vi "FloaterThreshAverage.vi"() -> ()   [LabVIEW 2022 SP3]
uses:
  <vilib>/Utility/file.llb/Read Delimited Spreadsheet (string).vi
panel:
  out "Array":string[][](array[string])
  in  "new path in":path=path "E:/Vitreous/CUMC/Single Element/SingleFloatersCompiled/AA_ThreshMaskResults.txt"
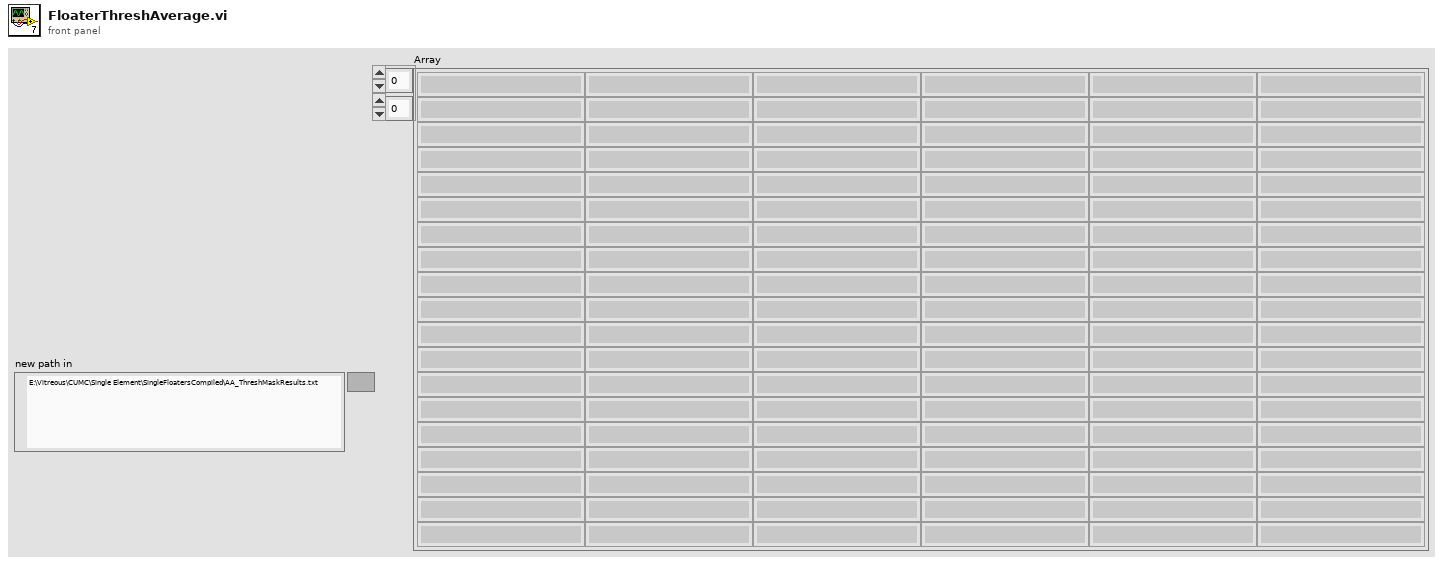
[diagram p1: front panel]
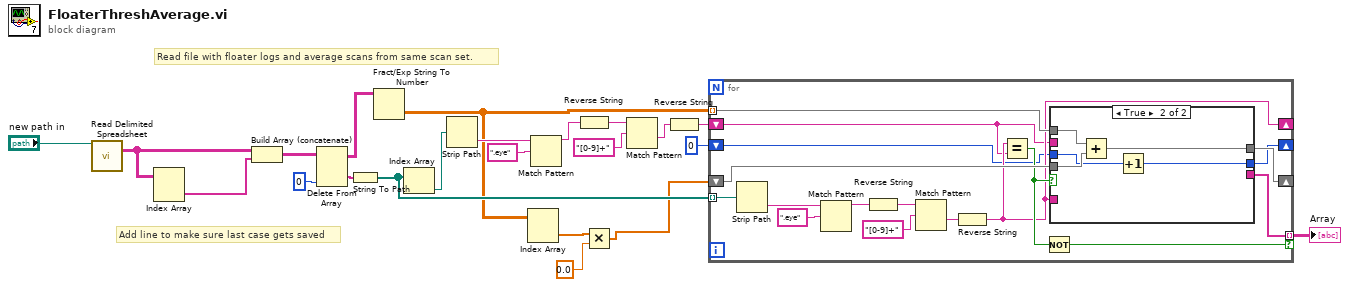
[diagram p0: block diagram]
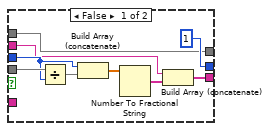
[diagram p2: hidden frame]
diagram:
  # "Read file with floater logs and average scans from same scan set."
  # "Add line to make sure last case gets saved"
  n1 = call-poly <vilib>:"Read Delimited Spreadsheet.vi"("file path (dialog if empty)"="new path in") -> ("all rows"=w2:string[][])  [unwired: 9 in, 5 out]
  n2 = Index Array(array=w2) -> (element=w1:string[])  [unwired: 2 in]
  n3 = Build Array (concatenate)(w2, w1) -> (w7:string[][])
  n4 = Delete From Array(array=w7, index (col)=0 ("index (row)")) -> (deleted portion=w8:string[], array with subset deleted=w20:string[][])  [unwired: 2 in]
  n5 = String To Path(string=w8) -> (path=w12:path[])
  n6 = Fract/Exp String To Number(string=w20) -> (number=w6:dbl[][])  [unwired: 3 in, 1 out]
  n7 = Index Array(array=w12) -> (element=w11:path)  [unwired: 1 in]
  n8 = Strip Path(path=w11) -> (name=w10:string)  [unwired: 1 out]
  n9 = Index Array(array=w6) -> (element=w5:dbl[])  [unwired: 2 in]
  n10 = Match Pattern(string=w10, regular expression=".eye") -> (before substring=w16:string)  [unwired: 1 in, 3 out]
  n11 = Reverse String(1:w16) -> (0:w15:string)
  n12 = Multiply(x=w5, y=0.0) -> (x*y=w4:dbl[])
  n13 = Match Pattern(string=w15, regular expression="[0-9]+") -> (after substring=w13:string)  [unwired: 1 in, 3 out]
  n14 = Reverse String(1:w13) -> (0:w9:string)
  n15 = for {
    tunnel: w12 -> [w39] mode=indexing
    shift-right: [w25] -> _
    shift-left: w9 -> [w23]
    tunnel: w6 -> [w32] mode=indexing
    shift-right: [w31] -> _
    shift-left: w4 -> [w30]
    shift-right: [w29] -> _
    shift-left: i16 0 -> [w24]
    tunnel: [w26] -> w18 mode=indexing if=w27
    n16 = Strip Path(path=w39) -> (name=w37:string)  [unwired: 1 out]
    n17 = Match Pattern(string=w37, regular expression=".eye") -> (before substring=w36:string)  [unwired: 1 in, 3 out]
    n18 = Reverse String(1:w36) -> (0:w35:string)
    n19 = Match Pattern(string=w35, regular expression="[0-9]+") -> (after substring=w33:string)  [unwired: 1 in, 3 out]
    n20 = Reverse String(1:w33) -> (0:w25:string)
    n21 = Equal?(x=w25, y=w23) -> (x = y?=w28:bool)
    n22 = Not(x=w28) -> (.not. x?=w27:bool)
    n23 = case shown="True" w28 {
      tunnel: w32 -> [w41 w53]
      tunnel: [w41 w52] -> w31
      tunnel: w30 -> [w48 w51]
      tunnel: [i16 1 w50] -> w29
      tunnel: w24 -> [w46 w49]
      tunnel: w25 -> [_ _]
      tunnel: [w42 _] -> w26
      tunnel: w23 -> [w40 _]
      frame False {
        n24 = Divide(x=w48, y=w46) -> (x/y=w45:dbl[])
        n25 = Build Array (concatenate)(w46, w45) -> (w44:dbl[])
        n26 = Number To Fractional String(number=w44) -> (F-format string=w43:string[])  [unwired: 3 in]
        n27 = Build Array (concatenate)(w40, w43) -> (w42:string[])
      }
      frame True {
        n28 = Add(x=w53, y=w51) -> (x+y=w52:dbl[])
        n29 = Increment(x=w49) -> (x+1=w50:i16)
      }
    }
  }
  "Array" <- w18
